vi "ALR scada init.vi"(8 "error in (no error)":errorcluster, 10 "N_param":i32, 11 "ALR_State in":T1) -> (0 "error out":errorcluster, 3 "ALR_State out":T1)   [LabVIEW 2019, in "Alarms.lvlib"]
uses:
  Alarms.lvlib
  Ctl/ALRs_State.ctl
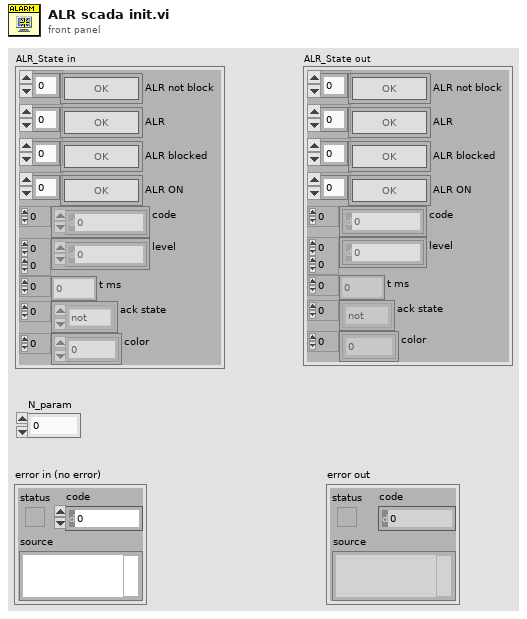
[diagram p1: front panel]
types:
  T1 = typedef "Alarms.lvlib/ALRs_State.ctl" = cluster{"ALR not block":bool[], "ALR":bool[], "ALR blocked":bool[], "ALR ON":bool[], "code":i32[], "level":i32[][], "t ms":u32[], "ack state":enum32{"not", "tripped", "reset", "ack"}[], "color":u32[]}
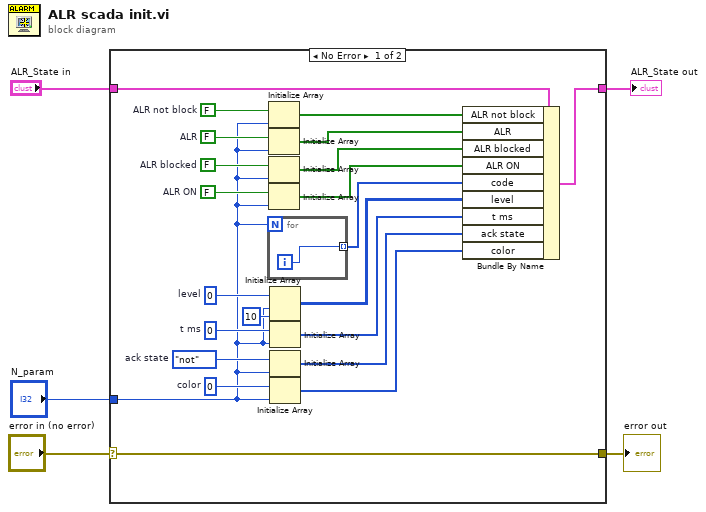
[diagram p0: block diagram]
diagram:
  n1 = case shown="No Error" "error in (no error)" {
    selector: "error in (no error)" -> [w6 w29]
    tunnel: [w7 w30] -> w2
    tunnel: "ALR_State in" -> [w8 w30]
    tunnel: "N_param" -> [w9 _]
    tunnel: [w6 w29] -> w3
    frame No Error {
      w11 = FALSE  # ALR not block
      w24 = u32 0  # color
      w23 = enum32{"not", "tripped", "reset", "ack"}."not"  # ack state
      w22 = u32 0  # t ms
      w21 = 0  # level
      w27 = FALSE  # ALR ON
      w26 = FALSE  # ALR blocked
      w25 = FALSE  # ALR
      n2 = for {
        N: w9 -> [_]
        tunnel: [w28] -> w16 mode=indexing
        i -> [w28]
      }
      n3 = Initialize Array(w11, w9) -> (w10:bool[])
      n4 = Initialize Array(w25, w9) -> (w19:bool[])
      n5 = Initialize Array(w26, w9) -> (w18:bool[])
      n6 = Initialize Array(w27, w9) -> (w17:bool[])
      n7 = Initialize Array(w21, w9, 10 ("dimension size")) -> (w15:i32[][])
      n8 = Initialize Array(w22, w9) -> (w14:u32[])
      n9 = Initialize Array(w23, w9) -> (w12:enum32{"not", "tripped", "reset", "ack"}[])
      n10 = Initialize Array(w24, w9) -> (w13:u32[])
      n11 = Bundle By Name(cluster=w8, "ALR not block"=w10, "ALR"=w19, "ALR blocked"=w18, "ALR ON"=w17, "code"=w16, "level"=w15, "t ms"=w14, "ack state"=w12, "color"=w13) -> (w7:T1)
    }
    frame Error {
    }
  }
  "error out" <- w3
  "ALR_State out" <- w2
